vi "Tutorial1.vi"() -> ()   [LabVIEW 2021]
doc: "This is an application which demonstrates some basic features of LabVIEW and the LINX package, through using a couple of buttons to turn and off the Arduino's built in LED, along with a pause option."
uses:
  <vilib>/MakerHub/LINX/Public/Peripherals/Digital/Digital Write 1 Chan.vi
  <vilib>/MakerHub/LINX/Public/Peripherals/Digital/Digital Write N Chans.vi
  <vilib>/MakerHub/LINX/Private/Local IO/LinxDigitalWrite.vi
  <vilib>/MakerHub/LINX/Public/Utilities/Check Channel.vi
  <vilib>/MakerHub/LINX/Public/Utilities/Open Serial.vi
  <vilib>/MakerHub/LINX/Private/Utilties/Generate Error.vi
  <vilib>/MakerHub/LINX/LMH-LINX.lvlib
panel:
  out "Boolean":bool
  in  "Pause":bool
  in  "Stop":bool
  in  "DO Channel":u8
  in  "Serial Port":refnum<visa-resource-name>="N/A"
  in  "Switch 2":bool
  in  "Switch 1":bool
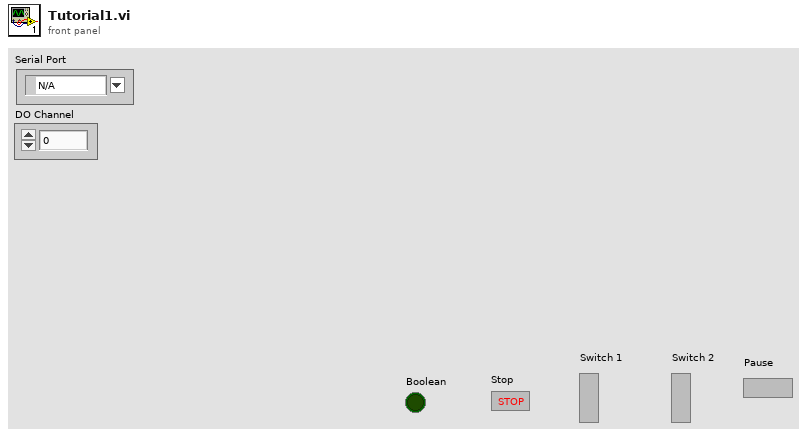
[diagram p1: front panel]
types:
  T1 = typedef "LMH-LINX.lvlib/LINX Ref.ctl" = cluster{"IO":T2, "Interface":T3, "LINX Device Config":T4}
  T2 = typedef "LMH-LINX.lvlib/Platform.ctl" = enum16{"Remote", "Local"}
  T3 = typedef "LMH-LINX.lvlib/Interface.ctl" = enum16{"Serial", "TCP"}
  T4 = typedef "LMH-LINX.lvlib/Device.lvlib/LINX Device Config.ctl" = cluster{"Interface":T3, "COM Port":refnum<visa-resource-name>, "TCP Configuration":T5, "Device Family":u8, "Device ID":u8, "Device Name":string, "TCP Ref":refnum<k5>, "Channels":T6}
  T5 = typedef "LMH-LINX.lvlib/Device.lvlib/TCP Config.ctl" = cluster{"IP Address":string, "Port":u16}
  T6 = typedef "LMH-LINX.lvlib/Channels.ctl" = cluster{"DI":u8[], "DO":u8[], "AI":u8[], "AO":u8[], "PWM":u8[], "QE":u8[], "UART":u8[], "I2C 2":u8[], "SPI":u8[], "CAN":u8[], "Servo":u8[], "AI Ref (V)":dbl, "AI Resolution (Bits)":u8, "AO Ref (V)":dbl, "AO Resolution (Bits)":u8}
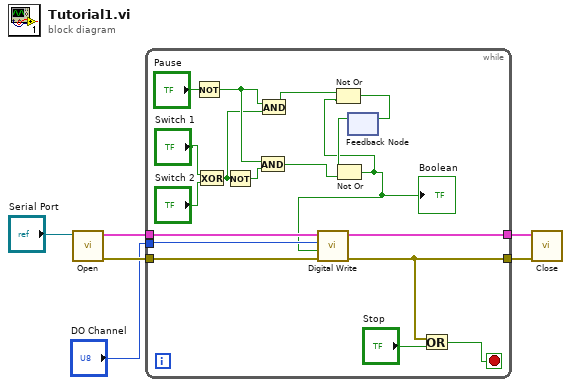
[diagram p0: block diagram]
diagram:
  n1 = call-poly <vilib>:"Open.vi"("Serial Port"="Serial Port") -> ("Error Out"=w4:errorcluster, "LINX Resource"=w6:T1)  [unwired: 8 in, 1 out]
  n2 = while {
    tunnel: w6 -> [w24]
    tunnel: [w23] -> w5
    tunnel: w4 -> [w22]
    tunnel: [w19] -> w3
    tunnel: "DO Channel" -> [w21]
    stop <- w18 stop-if-true
    n3 = Not(x="Pause") -> (.not. x?=w13:bool)
    n4 = Exclusive Or(1:"Switch 2", 2:"Switch 1") -> (0:w12:bool)
    n5 = Not(x=w12) -> (.not. x?=w14:bool)
    n6 = And(x=w13, y=w14) -> (x .and. y?=w10:bool)
    n7 = And(x=w13, y=w12) -> (x .and. y?=w11:bool)
    n8 = feedback #1() -> (w8:bool)  [unwired: 1 in]
    n9 = Not Or(1:w10, 2:w8) -> (0:w7:bool)
    "Boolean" <- w7
    n10 = call-poly <vilib>:"Digital Write.vi"("Error In"=w22, "Output Value"=w7, "DO Channel"=w21, "LINX Resource"=w24) -> ("Error Out"=w19:errorcluster, "LINX Resource"=w23:T1)  [unwired: 6 in]
    n11 = Not Or(1:w7, 2:w11) -> (0:w9:bool)
    n12 = feedback-in #1(w9) -> ()
    n13 = Or(x=w19, y="Stop") -> (x .or. y?=w18:bool)
  }
  n14 = call <vilib>:"Close.vi"("Error In"=w3, "LINX Resource"=w5) -> ()  [unwired: 9 in, 1 out]
